vi "Logout.vi"(0 "reference in":refnum<class "Login_Dialog.lvclass">, 5 "error in (no error)":errorcluster) -> (14 "reference in":refnum<class "Login_Dialog.lvclass">, 19 "error out":errorcluster)   [LabVIEW 2022 SP3, in "Login_Dialog.lvlib" / "Login_Dialog.lvclass"]
uses:
  Login_Dialog.lvclass
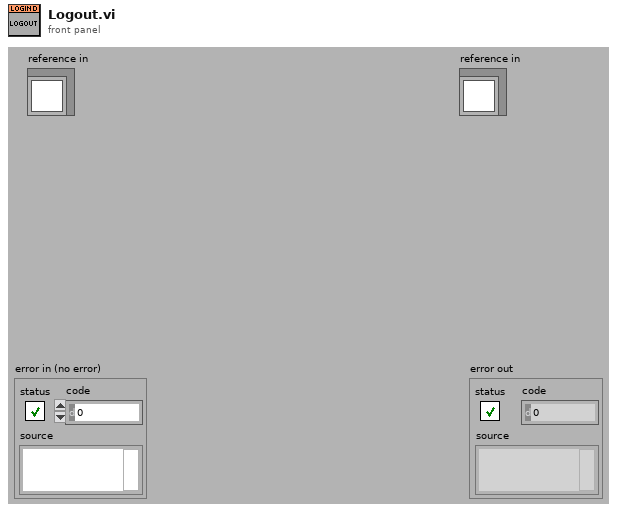
[diagram p1: front panel]
types:
  T1 = typedef "Login_Dialog.lvlib/Login_Dialog.lvclass/ObjectAttributes.ctl" = cluster{"Config":T2, "User":string, "LoggedIn":bool, "Users":string[][]}
  T2 = typedef "Login_Dialog.lvlib/Login_Dialog.lvclass/Config.ctl" = cluster{"default":string}
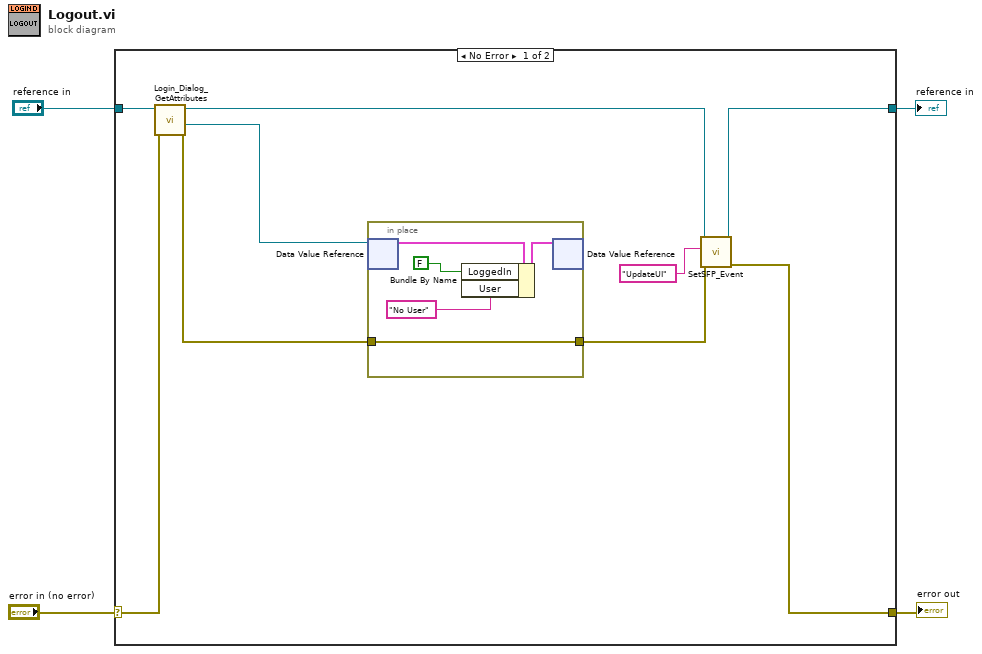
[diagram p0: block diagram]
diagram:
  n1 = case shown="No Error" "error in (no error)" {
    selector: "error in (no error)" -> [w13 w20]
    tunnel: [w9 w20] -> w3
    tunnel: [w5 w19] -> w1
    tunnel: "reference in" -> [w12 w19]
    frame No Error {
      n2 = call "Login_Dialog_GetAttributes.vi"("error in (no error)"=w13, "reference in"=w12) -> ("error out"=w10:errorcluster, "DataRef"=w11:refnum<data-value>, "reference out"=w6:refnum<class "Login_Dialog.lvclass">)  [unwired: 6 in, 1 out]
      n3 = in-place {
        in-place-border: [w15] -> w7
        in-place-border: w10 -> [w15]
        n4 = in-place-dvr #1(w11) -> (w18:T1)  [unwired: 1 out]
        n5 = Bundle By Name(cluster=w18, "LoggedIn"=FALSE, "User"="No User") -> (w17:T1)
        n6 = in-place-dvr #1(w17) -> ()  [unwired: 2 out]
      }
      n7 = call-dynamic "SetSFP_Event.vi"("error in (no error)"=w7, "msg"="UpdateUI", "reference in"=w6) -> ("error out"=w9:errorcluster, "reference out"=w5:refnum<class "Login_Dialog.lvclass">)  [unwired: 7 in]
    }
    frame Error {
    }
  }
  "error out" <- w3
  "reference in" <- w1
